vi "Ex1.vi"() -> ()   [LabVIEW 2016]
panel:
  out "주사위 6":dbl
  out "주사위 5":dbl
  out "주사위 4":dbl
  out "주사위 3":dbl
  out "주사위  2":dbl
  out "주사위 1":dbl
  out "주사위 랜덤":dbl[](array[numeric])
  in  "횟수":i32
  # "확률"
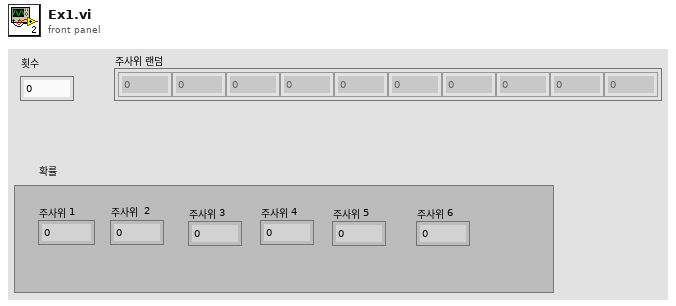
[diagram p1: front panel]
types:
  T1 = cluster{"주사위1":i32, "주사위 2":i32, "주사위 3":i32, "주사위 4":i32, "주사위 5":i32, "주사위 6":i32}
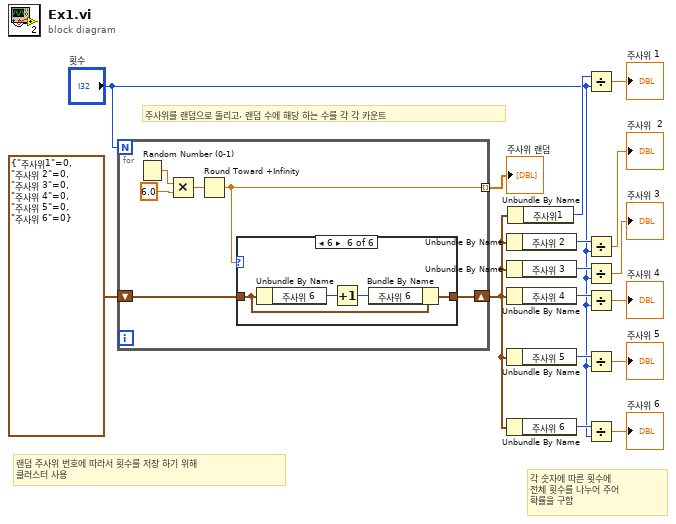
[diagram p0: block diagram]
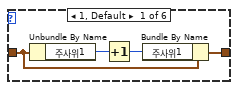
[diagram p2: hidden frame]
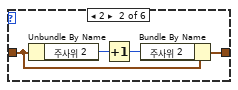
[diagram p3: hidden frame]
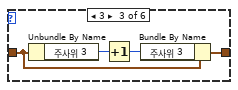
[diagram p4: hidden frame]
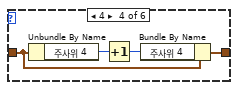
[diagram p5: hidden frame]
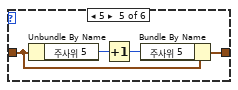
[diagram p6: hidden frame]
diagram:
  # "주사위를 랜덤으로 돌리고, 랜덤 수에 해당 하는 수를 각 각 카운트"
  # "각 숫자에 따른 횟수에 \n전체 횟수를 나누어 주어 \n확률을 구함"
  # "랜덤 주사위 번호에 따라서 횟수를 저장 하기 위해\n클러스터 사용"
  n1 = for {
    N: "횟수" -> [_]
    shift-right: [w18] -> w1
    shift-left: T1 {"주사위1"=0, "주사위 2"=0, "주사위 3"=0, "주사위 4"=0, "주사위 5"=0, "주사위 6"=0} -> [w19]
    tunnel: [w17] -> w15 mode=indexing
    n2 = Random Number (0-1)() -> (number: 0 to 1=w22:dbl)
    n3 = Multiply(x=w22, y=6.0) -> (x*y=w20:dbl)
    n4 = Round Toward +Infinity(x=w20) -> (ceil(x): smallest int >= x=w17:dbl)
    n5 = case shown="6" w17 {
      tunnel: w19 -> [w24 w28 w32 w36 w40 w44]
      tunnel: [w23 w27 w31 w35 w39 w43] -> w18
      frame 1, Default {
        n6 = Unbundle By Name(w24) -> ("주사위1"=w26:i32)
        n7 = Increment(x=w26) -> (x+1=w25:i32)
        n8 = Bundle By Name(cluster=w24, "주사위1"=w25) -> (w23:T1)
      }
      frame 2 {
        n9 = Unbundle By Name(w28) -> ("주사위 2"=w30:i32)
        n10 = Increment(x=w30) -> (x+1=w29:i32)
        n11 = Bundle By Name(cluster=w28, "주사위 2"=w29) -> (w27:T1)
      }
      frame 3 {
        n12 = Unbundle By Name(w32) -> ("주사위 3"=w34:i32)
        n13 = Increment(x=w34) -> (x+1=w33:i32)
        n14 = Bundle By Name(cluster=w32, "주사위 3"=w33) -> (w31:T1)
      }
      frame 4 {
        n15 = Unbundle By Name(w36) -> ("주사위 4"=w38:i32)
        n16 = Increment(x=w38) -> (x+1=w37:i32)
        n17 = Bundle By Name(cluster=w36, "주사위 4"=w37) -> (w35:T1)
      }
      frame 5 {
        n18 = Unbundle By Name(w40) -> ("주사위 5"=w42:i32)
        n19 = Increment(x=w42) -> (x+1=w41:i32)
        n20 = Bundle By Name(cluster=w40, "주사위 5"=w41) -> (w39:T1)
      }
      frame 6 {
        n21 = Unbundle By Name(w44) -> ("주사위 6"=w46:i32)
        n22 = Increment(x=w46) -> (x+1=w45:i32)
        n23 = Bundle By Name(cluster=w44, "주사위 6"=w45) -> (w43:T1)
      }
    }
  }
  "주사위 랜덤" <- w15
  n24 = Unbundle By Name(w1) -> ("주사위 2"=w12:i32)
  n25 = Unbundle By Name(w1) -> ("주사위 3"=w10:i32)
  n26 = Unbundle By Name(w1) -> ("주사위 4"=w8:i32)
  n27 = Unbundle By Name(w1) -> ("주사위 5"=w6:i32)
  n28 = Unbundle By Name(w1) -> ("주사위 6"=w4:i32)
  n29 = Unbundle By Name(w1) -> ("주사위1"=w14:i32)
  n30 = Divide(x=w14, y="횟수") -> (x/y=→"주사위 1":dbl)
  n31 = Divide(x=w12, y="횟수") -> (x/y=→"주사위  2":dbl)
  n32 = Divide(x=w10, y="횟수") -> (x/y=→"주사위 3":dbl)
  n33 = Divide(x=w8, y="횟수") -> (x/y=→"주사위 4":dbl)
  n34 = Divide(x=w6, y="횟수") -> (x/y=→"주사위 5":dbl)
  n35 = Divide(x=w4, y="횟수") -> (x/y=→"주사위 6":dbl)
